vi "TGT.vi"(0 "System no.":i32=1 min=1 max=4 step=1, 2 "Timing":i32=1 min=1 step=1, 5 "error in":errorcluster) -> (19 "error out":errorcluster)   [LabVIEW 2026]
doc: "Set trajectory timing. For further details, see Trajectories for Motion Paths in the controller user manual.\n\nC-867, C-884:"
panel:
  # "Set trajectory timing."
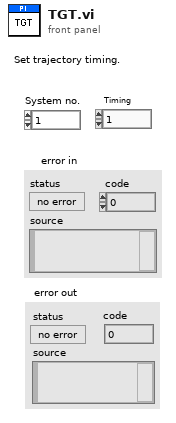
[diagram p1: front panel]
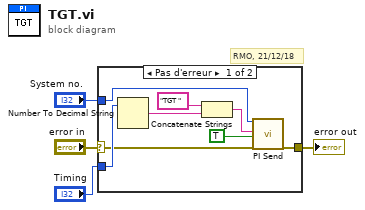
[diagram p0: block diagram]
diagram:
  # "RMO, 21/12/18"
  n1 = case shown="Pas d'erreur" "error in" {
    selector: "error in" -> [w5 w13]
    tunnel: [w12 w13] -> w4
    tunnel: "System no." -> [w11 _]
    tunnel: "Timing" -> [w10 _]
    frame No Error {
      n2 = Number To Decimal String(number=w10) -> (decimal integer string=w9:string)  [unwired: 1 out]
      n3 = Concatenate Strings("TGT ", w9) -> (w6:string)
      n4 = call "PI Send.vi"("System no."=w11, "String to send"=w6, "Attach termination char.?"=TRUE ("Attach Linefeed?"), "error in"=w5) -> ("error out"=w12:errorcluster)  [unwired: 2 in, 13 out]
    }
    frame Error {
    }
  }
  "error out" <- w4
